vi "Fetch.vi"(7 "Channel":i32(ring)=1 items=["Channel 1"=1, "Channel 2"=2, "Channel 3"=3, "Channel 4"=4, "Channel 5"=5, "Channel 6"=6, "Channel 7"=7, "Channel 8"=8, "Channel 8"=9, "Channel 10"=10, "Channel 11"=11, "Channel 12"=12, "Channel 13"=13, "Channel 14"=14, "Channel 15"=15, "Channel 16"=16], 8 "error in":errorcluster, 9 "Max Timeout(ms)":u32=10000, 10 "Fetch Type":u16(ring) items=["Current", "Power", "Voltage", "Capacity", "Temperature", "A-Hour", "W-Hour", "ACMeter EACTotal", "ACMeter EACStage"], 11 "VISA resource name":refnum<visa-resource-name>) -> (0 "error out":errorcluster, 2 "Measurement":dbl format="%.3g", 3 "VISA resource name out":refnum<visa-resource-name>)   [LabVIEW 2020, in "IT-M3400.lvlib"]
doc: "<b>Fetch Type</b>\n0:Current\n1:Power\n2:Voltage\n3:Capacity\n4:Temperature\n5:A-Hour\n6:W-Hour\n7:ACMeter EACTotal\n8:ACMeter EACStage"
uses:
  IT-M3400.lvlib
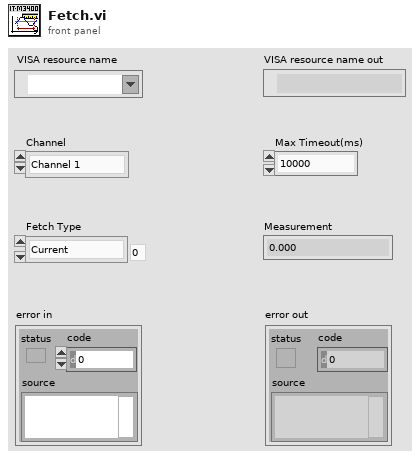
[diagram p1: front panel]
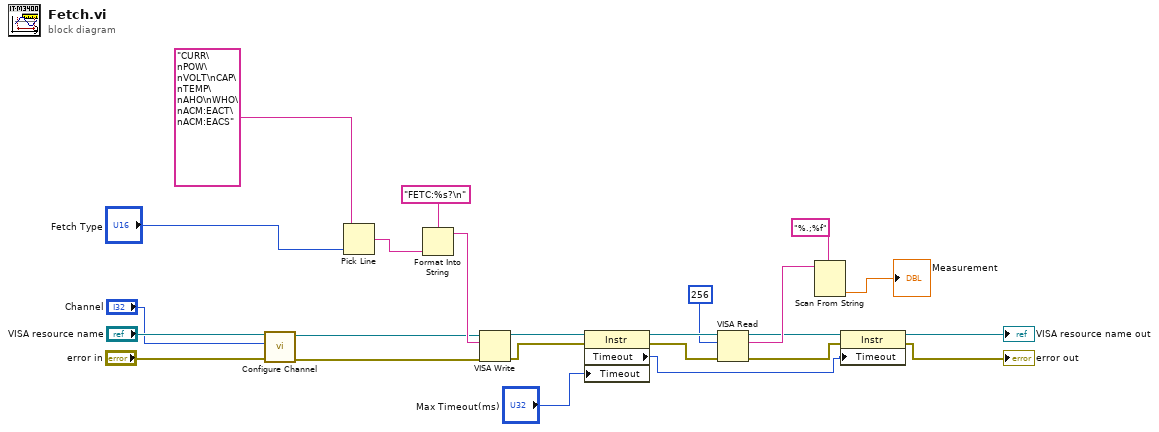
[diagram p0: block diagram]
diagram:
  n1 = call "Configure Channel.vi"("error in"="error in", "Channel"="Channel", "VISA resource name"="VISA resource name") -> ("error out"=w6:errorcluster, "VISA resource name out"=w7:refnum<visa-resource-name>)  [unwired: 7 in]
  n2 = Pick Line(multi-line string="CURR\nPOW\nVOLT\nCAP\nTEMP\nAHO\nWHO\nACM:EACT\nACM:EACS", line index="Fetch Type") -> (output string=w12:string)  [unwired: 1 in]
  n3 = Format Into String ("格式化写入字符串")(format string="FETC:%s?\n", w12) -> (resulting string=w23:string)  [unwired: 2 in, 1 out]
  n4 = VISA Write(VISA resource name=w7, write buffer=w23, error in (no error)=w6) -> (VISA resource name out=w10:refnum<visa-resource-name>, error out=w9:errorcluster)  [unwired: 1 out]
  n5 = property class="Instr"(reference=w10, error in=w9, "Timeout"="Max Timeout(ms)") -> (reference out=w20:refnum<visa-resource-name>, error out=w19:errorcluster, "Timeout"=w8:u32)
  n6 = VISA Read(VISA resource name=w20, byte count=256, error in (no error)=w19) -> (VISA resource name out=w16:refnum<visa-resource-name>, read buffer=w22:string, error out=w11:errorcluster)  [unwired: 1 out]
  n7 = Scan From String(format string="%.;%f", input string=w22) -> (output 1=→"Measurement":dbl)  [unwired: 3 in, 3 out]
  n8 = property class="Instr"(reference=w16, error in=w11, "Timeout"=w8) -> (reference out=→"VISA resource name out":refnum<visa-resource-name>, error out=→"error out":errorcluster)
